vi "表格颜色-8.6.vi"(6 "列数?":bool, 8 "颜色类型":u32[](array[colorbox]), 9 "列数":i32=2, 10 "行数":i32=13, 11 "表格引用":refnum<vi>) -> ()   [LabVIEW 2013]
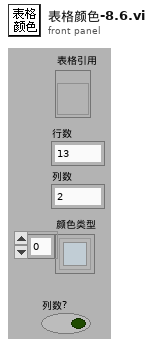
[diagram p1: front panel]
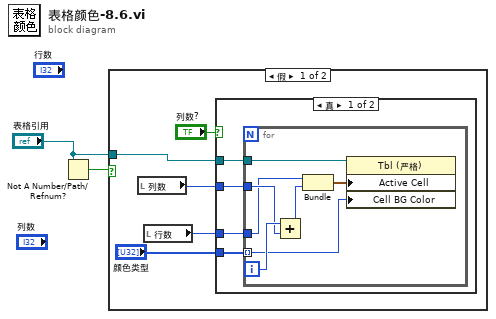
[diagram p0: block diagram]
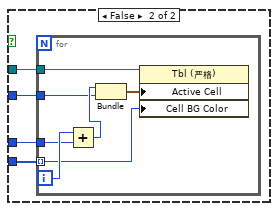
[diagram p2: hidden frame]
diagram:
  n1 = Not A Number/Path/Refnum?(number/path/refnum="表格引用") -> (NaN/Path/Refnum?=w2:bool)
  n2 = case shown="假" w2 {
    tunnel: "表格引用" -> [w7 _]
    frame False {
      n3 = local read "列数"() -> (w4:i32)
      n4 = local read "行数"() -> (w5:i32)
      n5 = case shown="真" "列数?" {
        tunnel: w7 -> [w11 w22]
        tunnel: "颜色类型" -> [w10 w21]
        tunnel: w5 -> [w9 w20]
        tunnel: w4 -> [w8 w19]
        frame True {
          n6 = for {
            tunnel: w11 -> [w18]
            tunnel: w10 -> [w15] mode=indexing
            tunnel: w9 -> [w12]
            tunnel: w8 -> [w14]
            i -> [w16]
            n7 = Add(x=w16, y=w14) -> (x+y=w13:i32)
            n8 = Bundle("行数"=w12, w13) -> (w17:cluster{"行数":i32, i32})  [unwired: 1 out]
            n9 = property class="Tbl (严格)"(reference=w18, "Active Cell"=w17, "Cell BG Color"=w15) -> ()  [unwired: 1 in, 2 out]
          }
        }
        frame False {
          n10 = for {
            tunnel: w22 -> [w29]
            tunnel: w21 -> [w26] mode=indexing
            tunnel: w20 -> [w25]
            tunnel: w19 -> [w23]
            i -> [w27]
            n11 = Add(x=w27, y=w25) -> (x+y=w24:i32)
            n12 = Bundle(w24, "列数"=w23) -> (w28:cluster{i32, "列数":i32})  [unwired: 1 out]
            n13 = property class="Tbl (严格)"(reference=w29, "Active Cell"=w28, "Cell BG Color"=w26) -> ()  [unwired: 1 in, 2 out]
          }
        }
      }
    }
    frame True {
    }
  }
